vi "Calibrate Ticks 2 Temperature (uSMC).vi"(1 "SMindex":i32, 2 "temperature (ticks)":u16) -> (0 "Temperature (Cels)":dbl)   [LabVIEW 2010, in "SignalWriterMH110203USBStepperMotor.lvclass"]
uses:
  SignalWriterMH110203USBStepperMotor.lvclass
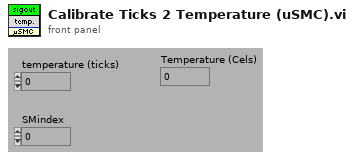
[diagram p1: front panel]
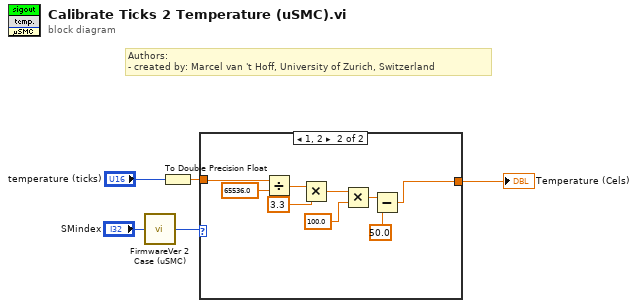
[diagram p0: block diagram]
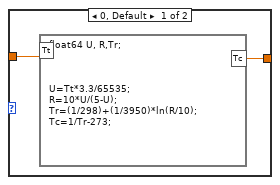
[diagram p2: hidden frame]
diagram:
  # "Authors: \n- created by: Marcel van 't Hoff, University of Zurich, Switzerland"
  n1 = call "FirmwareVer 2 Case (uSMC).vi"("SMindex"="SMindex") -> ("Case"=w1:i32)
  n2 = To Double Precision Float(number="temperature (ticks)") -> (double precision float=w2:dbl)
  n3 = case shown="1, 2" w1 {
    tunnel: [w7 w8] -> w5
    tunnel: w2 -> [w6 w16]
    frame 0, Default {
      n4 = formula code="float64 U, R,Tr;\n\n\n\nU=Tt*3.3/65535;\nR=10*U/(5-U);\nTr=(1/298)+(1/3950)*ln(R/10);\nTc=1/Tr-273;"("Tt"=w6) -> ("Tc"=w7:dbl)
    }
    frame 1, 2 {
      n5 = Divide(x=w16, y=65536.0) -> (x/y=w14:dbl)
      n6 = Multiply(x=w14, y=3.3) -> (x*y=w12:dbl)
      n7 = Multiply(x=w12, y=100.0) -> (x*y=w10:dbl)
      n8 = Subtract(x=w10, y=50.0) -> (x-y=w8:dbl)
    }
  }
  "Temperature (Cels)" <- w5
